vi "Send Send Status Update.vi"(7 "Priority":T2=enum."Normal" caption="Message Priority (Normal)", 8 "error in (no error)":errorcluster, 9 "Status":T1=enum."Added", 10 "Task Name":string, 11 "Message Enqueuer in":refnum<class "Message Enqueuer.lvclass">) -> (0 "error out":errorcluster, 3 "Message Enqueuer out":refnum<class "Message Enqueuer.lvclass">)   [LabVIEW 2017, in "BuildWorker.lvlib" / "Send Status Update Msg.lvclass"]
doc: "Sends the <b>Send Status Update Msg.lvclass</b> message.\n\nThis message will call <b>Send Status Update.vi</b> on the <b>BuildWorker.lvlib:BuildWorker.lvclass</b> actor.\n\n<b>Send Status Update.vi Description</b>"
uses:
  Send Status Update Msg.lvclass
  <vilib>/ActorFramework/Message Enqueuer/Message Enqueuer.lvclass
  <vilib>/ActorFramework/Message Enqueuer/Message Priority.ctl
  Classes/Task Interface/Task/Status.ctl
  Applications/National Instruments/LabVIEW 2017 64-bit/vi.lib/ActorFramework/Message/Message.lvclass
  Send Status Update Msg.lvclass/Send Status Update Msg.ctl
  <vilib>/ActorFramework/Message Enqueuer/Message Enqueuer.lvclass/Message Enqueuer.ctl
  <vilib>/ActorFramework/Message Priority Queue/Priority Enqueue.vi
  Classes/Task Interface/Task/Task.lvclass
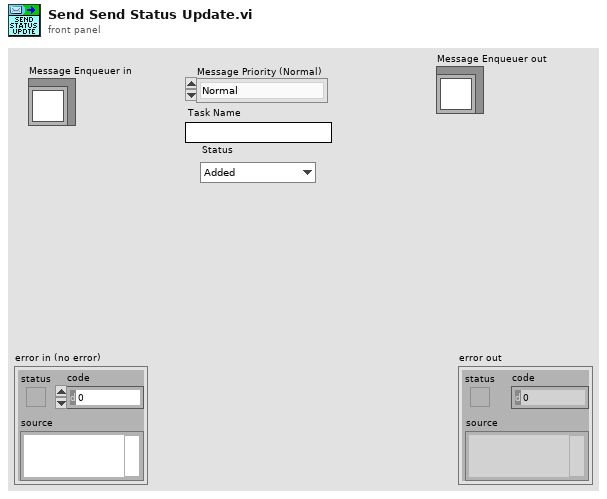
[diagram p1: front panel]
types:
  T1 = typedef "Task Interface.lvlib/Task.lvclass/Status.ctl" = enum16{"Created", "Added", "Pending", "Queued", "Processing", "Cleaning", "Building", "Finished", "Failed", "Removed", "Not found"}
  T2 = typedef "Actor Framework.lvlib/Message Enqueuer.lvclass/Message Priority.ctl" = enum16{"Low", "Normal", "High"}
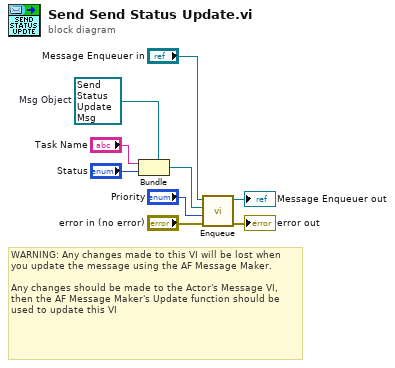
[diagram p0: block diagram]
diagram:
  w7 = refnum<class "Send Status Update Msg.lvclass"> refnum  # Msg Object
  # "WARNING: Any changes made to this VI will be lost when you update the message using the AF Message Maker.\n\nAny changes should be made to the Actor's Message VI, then the AF Message Maker's Update function should be used to update this VI"
  n1 = Bundle(cluster=w7, "Task Name", "Status") -> (w2:refnum<class "Send Status Update Msg.lvclass">)
  n2 = call <vilib>:"Enqueue.vi"("error in (no error)"="error in (no error)", "Message Priority (Normal)"="Priority", "Message"=w2, "Message Enqueuer in"="Message Enqueuer in") -> ("error out"=→"error out":errorcluster, "Message Enqueuer out"=→"Message Enqueuer out":refnum<class "Message Enqueuer.lvclass">)  [unwired: 6 in]
